vi "RT_interface.vi"() -> ()   [LabVIEW 2019]
uses:
  <vilib>/Platform/TimedLoop/XDataNode/timing_clust.ctl
  <vilib>/Platform/TimedLoop/XDataNode/nitl_modes.ctl
  <vilib>/Platform/TimedLoop/XDataNode/wakeup.ctl
  <vilib>/FPGAPlugInAG/myRIO-1900/niLvFpga_Open_myRIO-1900.vi
  <vilib>/rvi/interface/common/dynamic/niFpgaDynamicAddResources.vi
  <vilib>/Utility/error.llb/Error Cluster From Error Code.vi
  <vilib>/rvi/errors/niLvFpgaAdjustHostInterfaceError.vi
  <vilib>/FPGAPlugInAG/Dynamic/niLvFpga_Close_Dynamic.vi
  <vilib>/platform/TimedLoop/XDataNode/XDataNode.xnode
  <vilib>/rvi/interface/nirviOpenFPGA/nirviOpenFPGA.xnode
  FPGA Bitfiles/steeringandfeedi_FPGATarget_FPGAdriver_UwAVMcVyVAU.lvbitx
  <vilib>/rvi/interface/nirviReadWriteControl/nirviReadWriteControl.xnode
  <vilib>/rvi/interface/nirviCloseFPGA/nirviCloseFPGA.xnode
  <vilib>/Platform/TimedLoop/XDataNode/XDNodeRunTimeDep.lvlib
  <vilib>/rvi/interface/Simulation/niFpgaSimulationCallBeginRW.vi
  NiFpgaLv.dll
panel:
  out "Feed Reset":bool
  out "Steer Reset":bool
  out "Num Cycle":u32
  out "Duty Ratio":dbl
  out "stepper position":i32(graph)=-58
  out "PWM coil":dbl(graph)
  in  "Steering gain":dbl=1.0
  in  "Pushing Gain(-1)":dbl=-0.5
  in  "Enable stepper?":bool=TRUE
  out "Encoder 2 reading":i16(graph)=-924
  out "Encoder 1 reading":i16(graph)=-115
  out "Encoder1  Position":i16=-115
  in  "stop":bool
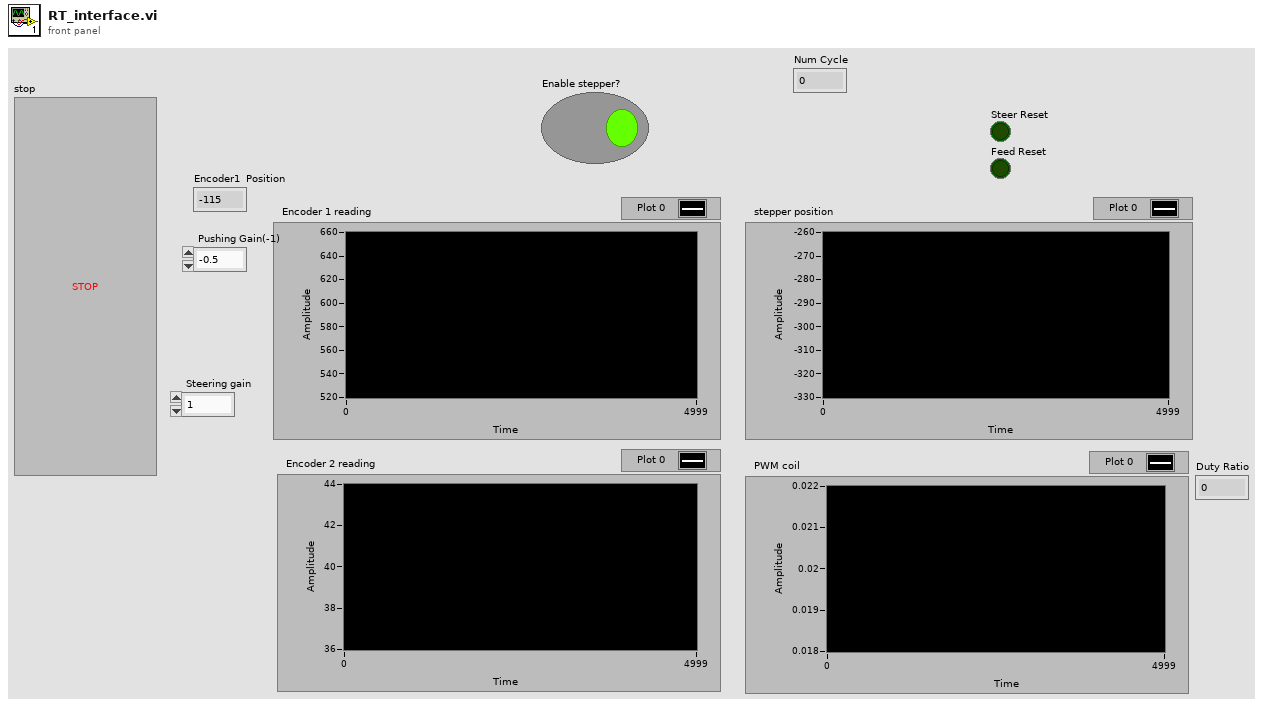
[diagram p1: front panel]
types:
  T1 = typedef "XDNodeRunTimeDep.lvlib/timing_clust.ctl" = cluster{"Expected End [f-1]":u64, "Actual End [f-1]":u64, "Finished Late? [f-1]":bool, "Expected End [i-1]":u64, "Actual End [i-1]":u64, "Finished Late? [i-1]":bool, "Expected Start [i]":u64, "Actual Start [i]":u64, "Expected Start [f]":u64, "Actual Start [f]":u64, "Source Name":string, "Structure Name":string, "Period":i64, "Deadline":i64, "Offset":i64, "Start":i64, "Priority":i32, "Timeout":i32, "Mode":T2, "Wakeup Reason":T3, "Error":errorcluster, "Source Type":string, "Secondary Source Type":string, "Global End Time":u64, "Global Start Time":u64, "Frame Duration":u64, "Iteration Duration":u64, "Assigned CPU":i32, "I/O Scan Engine Mode":u32}
  T2 = typedef "XDNodeRunTimeDep.lvlib/nitl_modes.ctl" = enum32{"No Change", "Process missed periods, maintain original phase", "Discard missed periods, maintain original phase", "Process missed periods, ignore original phase", "Discard missed periods, ignore original phase"}
  T3 = typedef "XDNodeRunTimeDep.lvlib/wakeup.ctl" = enum32{"Normal", "Aborted", "Asynchronous wakeup", "Timing source error", "Timed loop error", "Timeout"}
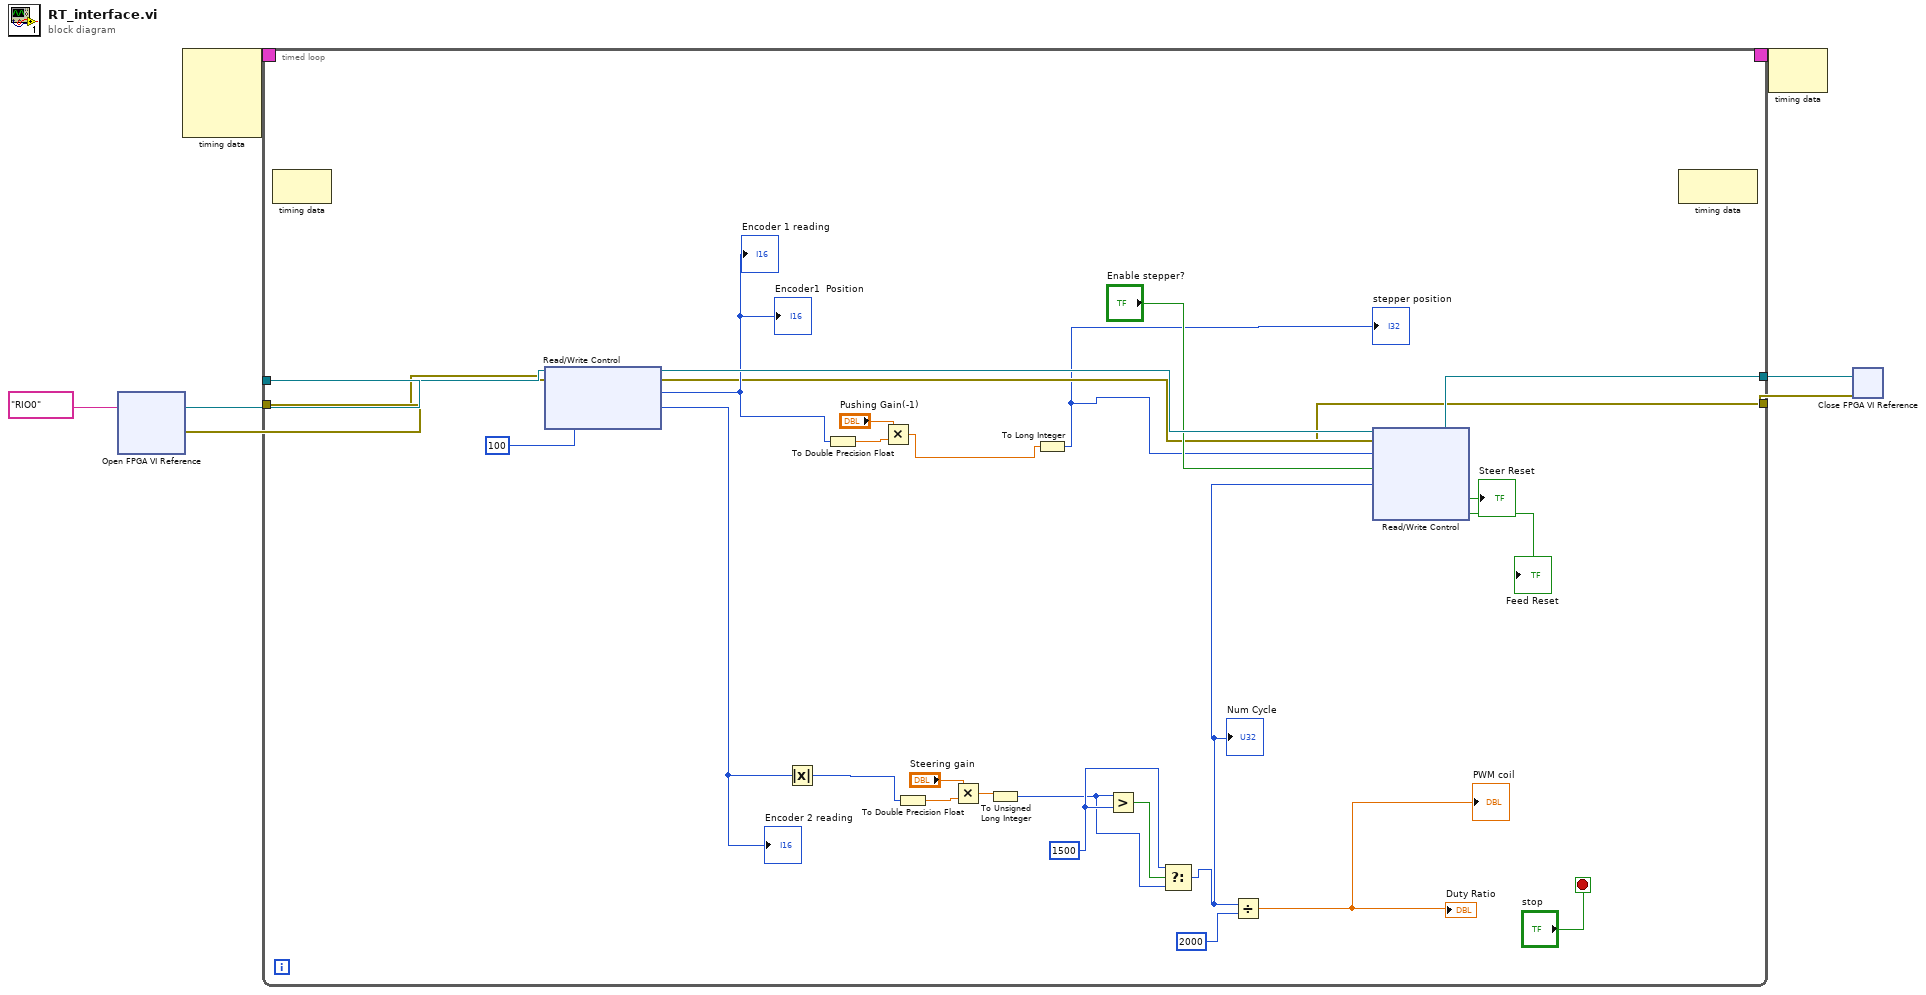
[diagram p0: block diagram]
diagram:
  n1 = xnode "Open FPGA VI Reference"("resource name"=tag "RIO0") -> ("FPGA VI Reference Out"=w5:refnum<k20>, "error out"=w4:errorcluster)  [unwired: 1 in]
  n2 = node-c288() -> (w7:T1)  [unwired: 4 in]
  n3 = timed-loop {
    timing: w7 -> [_]
    timing-out: [_] -> w6
    tunnel: w5 -> [w21]
    tunnel: w4 -> [w20]
    tunnel: [w32] -> w3
    tunnel: [w17] -> w2
    stop <- "stop" stop-if-true
    w23 = u32 1500 ("y")
    n4 = node-c288() -> ()  [unwired: 1 in, 1 out]
    n5 = xnode "Read/Write Control"("FPGA VI Reference In"=w21, "error in"=w20, "Velocity  Limit"=100) -> ("FPGA VI Reference Out"=w33:refnum<k20>, "error out"=w19:errorcluster, "Encoder Position"=w30:i16, "Encoder Position 2"=w12:i16)
    "Encoder1  Position" <- w30
    "Encoder 1 reading" <- w30
    "Encoder 2 reading" <- w12
    n6 = Absolute Value(x=w12) -> (abs(x)=w15:i16)
    n7 = To Double Precision Float(number=w30) -> (double precision float=w29:dbl)
    n8 = Multiply(x="Pushing Gain(-1)", y=w29) -> (x*y=w11:dbl)
    n9 = To Double Precision Float(number=w15) -> (double precision float=w26:dbl)
    n10 = Multiply(x="Steering gain", y=w26) -> (x*y=w25:dbl)
    n11 = To Unsigned Long Integer(number=w25) -> (unsigned 32bit integer=w13:u32)
    n12 = To Long Integer(number=w11) -> (32bit integer=w16:i32)
    "stepper position" <- w16
    n13 = Greater?(x=w13, y=w23) -> (0:w24:bool)
    n14 = Select(t=w23, s=w24, f=w13) -> (s? t:f=w10:u32)
    "Num Cycle" <- w10
    n15 = Divide(x=w10, y=u32 2000) -> (x/y=→"PWM coil" →"Duty Ratio":dbl)
    n16 = xnode "Read/Write Control"("FPGA VI Reference In"=w33, "error in"=w19, "Position Ref."=w16, "enable?"="Enable stepper?", "Num_cycle_on"=w10) -> ("FPGA VI Reference Out"=w32:refnum<k20>, "error out"=w17:errorcluster, "Steer Reset"=→"Steer Reset":bool, "Feed Reset"=→"Feed Reset":bool)
    n17 = node-c288() -> ()  [unwired: 1 in, 1 out]
  }
  n18 = node-c288(w6) -> ()  [unwired: 1 out]
  n19 = xnode "Close FPGA VI Reference"("FPGA VI Reference In"=w3, "error in"=w2) -> ()  [unwired: 1 out]
